vi "UIStep Setting Panel.vi"(8 "error in (no error)":errorcluster, 9 "Project In":refnum<class "Project.lvclass">, 11 "Step in":refnum<class "Step.lvclass">) -> (0 "error out":errorcluster, 3 "Step out":refnum<class "Step.lvclass">)   [LabVIEW 2015, in "UIStep.lvclass"]
uses:
  UIStep.lvclass
  Step.lvclass
  Project.lvclass
  SerializableObject/CONFIGURE_UI_STATE.ctl
  Editor/Editor.lvclass
panel:
  in  "Size":enum16{"Small", "Middle", "Big"}(ring)
  in  "Embedded":bool
  in  "Title":string
  in  "Text Content":string
  in  "Text Style":T1={"Font"="", "Size"=0.0, "Justification"=1, "TextColor"=0, "BGColor"=0, "Bold"=FALSE} {"Justification" items=["Left", "Center", "Right"]}
  in  "Buttons":T2
  in  "Image":path
  in  "Enable Input":bool
  in  "Input Validation":string caption="Input Validation(Regular Expression)"
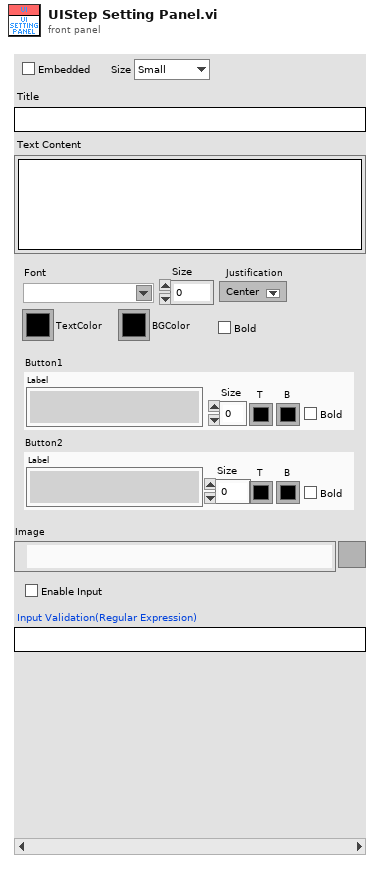
[diagram p1: front panel]
types:
  T1 = cluster{"Font":string, "Size":dbl, "Justification":u16, "TextColor":u32, "BGColor":u32, "Bold":bool}
  T2 = cluster{"Button1":cluster{"Label":string, "Size":dbl, "TextColor":u32, "BGColor":u32, "Bold":bool}, "Button2":cluster{"Label":string, "Size":dbl, "TextColor":u32, "BGColor":u32, "Bold":bool}}
  T3 = typedef "Editor.lvclass/CONFIGURE_UI_STATE.ctl" = enum16{"UI_LOOP", "INIT", "END", "CHANGE_PANEL"}
  T4 = enum8{"Enabled", "Disabled", "Disabled and Grayed Out"}
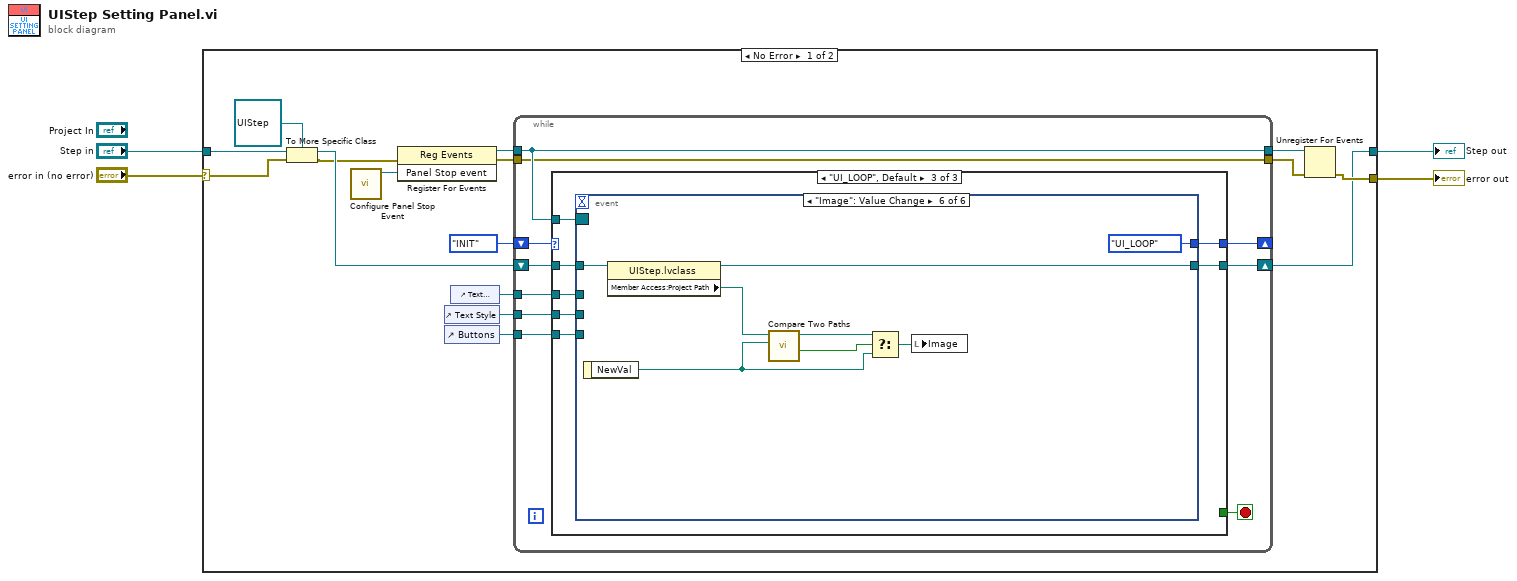
[diagram p0: block diagram]
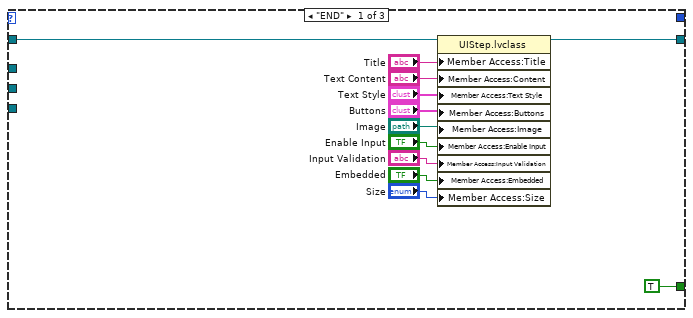
[diagram p2: hidden frame]
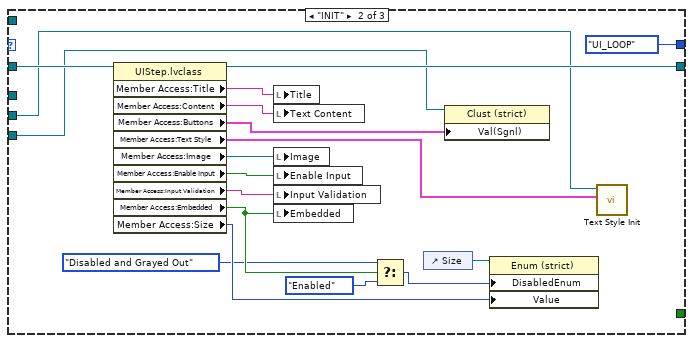
[diagram p3: hidden frame]
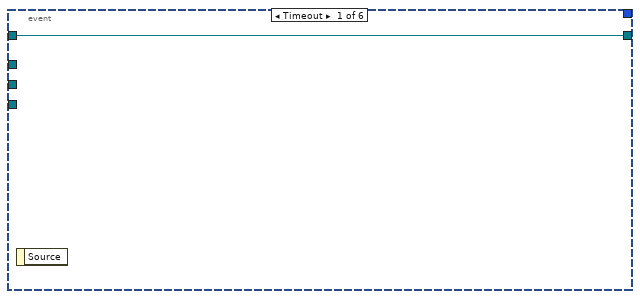
[diagram p4: hidden frame]
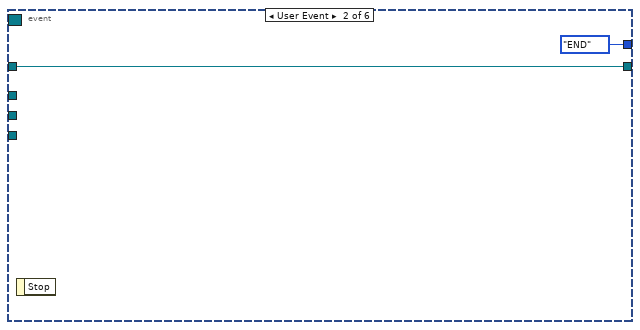
[diagram p5: hidden frame]
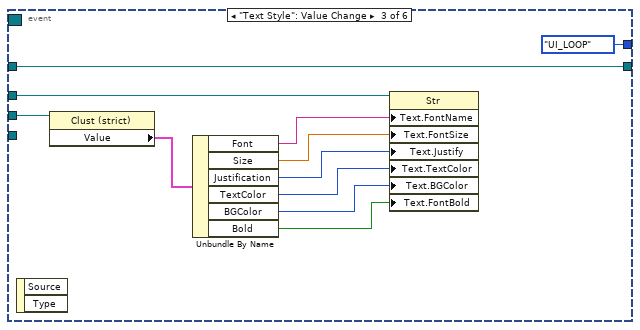
[diagram p6: hidden frame]
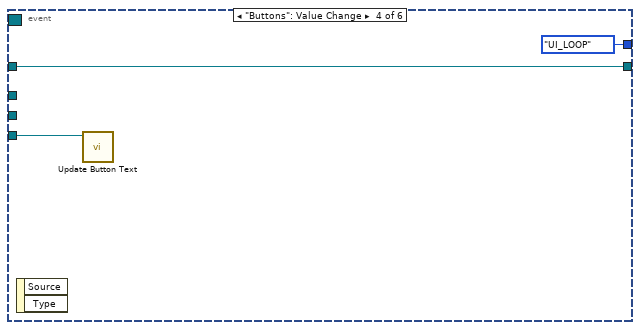
[diagram p7: hidden frame]
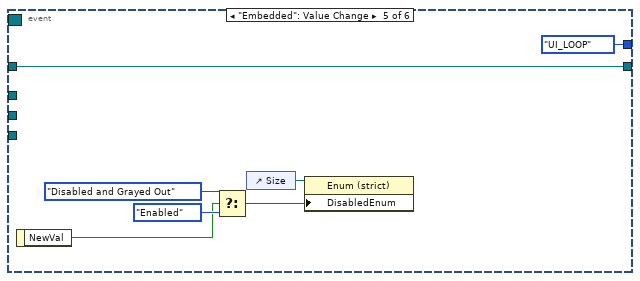
[diagram p8: hidden frame]
diagram:
  n1 = case shown="No Error" "error in (no error)" {
    selector: "error in (no error)" -> [w18 w101]
    tunnel: [w12 w101] -> w3
    tunnel: "Step in" -> [w20 w100]
    tunnel: [w11 w100] -> w1
    frame No Error {
      n2 = To More Specific Class(target class=refnum<class "UIStep.lvclass"> refnum ("ConfigureableObject in"), reference=w20, error in=w18) -> (specific class reference=w10:refnum<class "UIStep.lvclass">, error out=w9:errorcluster)
      n3 = call "Configure Panel Stop Event.vi"() -> ("Panel Stop event"=w5:refnum<user-event>)  [unwired: 11 in]
      n4 = register-events(error in=w9, w5) -> (reference out=w13:refnum<event-registration>, error out=w15:errorcluster)  [unwired: 1 in]
      n5 = control-ref of="Text Style"() -> (w8:refnum<vi>)
      n6 = control-ref of="Buttons"() -> (w6:refnum<vi>)
      n7 = control-ref of="Text Content"() -> (w7:refnum<vi>)
      n8 = while {
        tunnel: w13 -> [w30]
        tunnel: [w30] -> w14
        tunnel: w15 -> [w29]
        tunnel: [w29] -> w16
        shift-right: [w27] -> w11
        shift-left: w10 -> [w28]
        shift-right: [w25] -> _
        shift-left: CONFIGURE_UI_STATE."INIT" -> [w26]
        tunnel: w8 -> [w23]
        tunnel: w7 -> [w22]
        tunnel: w6 -> [w21]
        stop <- w24 stop-if-true
        n9 = case shown="\"UI_LOOP\", Default" w26 {
          tunnel: w30 -> [_ _ w67]
          tunnel: w28 -> [w41 w59 w66]
          tunnel: [w40 w58 w65] -> w27
          tunnel: [_ CONFIGURE_UI_STATE."UI_LOOP" w64] -> w25
          tunnel: [TRUE _ _] -> w24
          tunnel: w23 -> [_ w50 w63]
          tunnel: w22 -> [_ _ w62]
          tunnel: w21 -> [_ w52 w61]
          frame "END" {
            n10 = property class="UIStep.lvclass"(reference=w41, "Member Access:Title"="Title", "Member Access:Content"="Text Content", "Member Access:Text Style"="Text Style", "Member Access:Buttons"="Buttons", "Member Access:Image"="Image", "Member Access:Enable Input"="Enable Input", "Member Access:Input Validation"="Input Validation", "Member Access:Embedded"="Embedded", "Member Access:Size"="Size") -> (reference out=w40:refnum<class "UIStep.lvclass">)  [unwired: 1 in, 1 out]
          }
          frame "INIT" {
            n11 = property class="UIStep.lvclass"(reference=w59) -> (reference out=w58:refnum<class "UIStep.lvclass">, "Member Access:Title"=w57:string, "Member Access:Content"=w56:string, "Member Access:Buttons"=w51:T2, "Member Access:Text Style"=w49:T1, "Member Access:Image"=w55:path, "Member Access:Enable Input"=w54:bool, "Member Access:Input Validation"=w53:string, "Member Access:Embedded"=w47:bool, "Member Access:Size"=w48:enum16{"Small", "Middle", "Big"})  [unwired: 1 in, 1 out]
            n12 = local write "Title"(w57) -> ()
            n13 = local write "Text Content"(w56) -> ()
            n14 = local write "Image"(w55) -> ()
            n15 = local write "Enable Input"(w54) -> ()
            n16 = local write "Input Validation"(w53) -> ()
            n17 = local write "Embedded"(w47) -> ()
            n18 = Select(t=T4."Disabled and Grayed Out" ("Disabled"), s=w47, f=T4."Enabled" ("Disabled")) -> (s? t:f=w45:T4)
            n19 = control-ref of="Size"() -> (w43:refnum<vi>)
            n20 = property class="Clust (strict)"(reference=w52, "Val(Sgnl)"=w51) -> ()  [unwired: 1 in, 2 out]
            n21 = property class="Enum (strict)"(reference=w43, "DisabledEnum"=w45, "Value"=w48) -> ()  [unwired: 1 in, 2 out]
            n22 = call "Text Style Init.vi"("Text Style Value"=w49, "Text Style Ctrl"=w50) -> ()  [unwired: 10 in]
          }
          frame "UI_LOOP", Default {
            n23 = event shown="[5] \"Image\": Value Change" {
              selector: w67 -> [_ _ _ _ _ _]
              dyn-events: _ -> [_ _ _ _ _ _]
              timeout: _ -> [_ _ _ _ _ _]
              tunnel: w66 -> [w68 w70 w81 w84 w86 w99]
              tunnel: [w68 w70 w81 w84 w86 w94] -> w65
              tunnel: [_ CONFIGURE_UI_STATE."END" CONFIGURE_UI_STATE."UI_LOOP" CONFIGURE_UI_STATE."UI_LOOP" CONFIGURE_UI_STATE."UI_LOOP" CONFIGURE_UI_STATE."UI_LOOP"] -> w64
              tunnel: w63 -> [_ _ w79 _ _ _]
              tunnel: w62 -> [_ _ w78 _ _ _]
              tunnel: w61 -> [_ _ _ w82 _ _]
              event Timeout {
                n24 = event-data() -> ()  [unwired: 1 in, 1 out]
              }
              event User Event {
                n25 = event-data() -> ()  [unwired: 1 in, 1 out]
              }
              event "Text Style": Value Change {
                n26 = event-data() -> ()  [unwired: 1 in, 2 out]
                n27 = property class="Clust (strict)"(reference=w79) -> ("Value"=w77:T1)  [unwired: 1 in, 2 out]
                n28 = Unbundle By Name(w77) -> ("Font"=w76:string, "Size"=w75:dbl, "Justification"=w74:u16, "TextColor"=w73:u32, "BGColor"=w72:u32, "Bold"=w71:bool)
                n29 = property class="Str"(reference=w78, "Text.FontName"=w76, "Text.FontSize"=w75, "Text.Justify"=w74, "Text.TextColor"=w73, "Text.BGColor"=w72, "Text.FontBold"=w71) -> ()  [unwired: 1 in, 2 out]
              }
              event "Buttons": Value Change {
                n30 = event-data() -> ()  [unwired: 1 in, 2 out]
                n31 = call "Update Button Text.vi"("Buttons"=w82) -> ()  [unwired: 11 in]
              }
              event "Embedded": Value Change {
                n32 = event-data() -> ("NewVal"=w88:bool)  [unwired: 1 in]
                n33 = Select(t=T4."Disabled and Grayed Out" ("Disabled"), s=w88, f=T4."Enabled" ("Disabled")) -> (s? t:f=w91:T4)
                n34 = control-ref of="Size"() -> (w87:refnum<vi>)
                n35 = property class="Enum (strict)"(reference=w87, "DisabledEnum"=w91) -> ()  [unwired: 1 in, 2 out]
              }
              event "Image": Value Change {
                n36 = event-data() -> ("NewVal"=w95:path)  [unwired: 1 in]
                n37 = property class="UIStep.lvclass"(reference=w99) -> (reference out=w94:refnum<class "UIStep.lvclass">, "Member Access:Project Path"=w96:path)  [unwired: 1 in, 1 out]
                n38 = call <vilib>:"Compare Two Paths.vi"("Path 2"=w95, "Path 1"=w96) -> ("Path 2 Relative to Path 1?"=w97:bool, "Relative Path from 1 to 2"=w98:path)  [unwired: 6 in, 2 out]
                n39 = Select(t=w98, s=w97, f=w95) -> (s? t:f=w92:path)
                n40 = local write "Image"(w92) -> ()
              }
            }
          }
        }
      }
      n41 = Unregister For Events(event registration refnum=w14, error in=w16) -> (error out=w12:errorcluster)
    }
    frame Error {
    }
  }
  "error out" <- w3
  "Step out" <- w1
